vi "caluculator event structure.vi"() -> ()   [LabVIEW 2018]
panel:
  in  "stop":bool
  out "x/y":dbl
  out "x*y":dbl
  out "x-y":dbl
  out "C":dbl
  in  "B":dbl
  in  "A":dbl
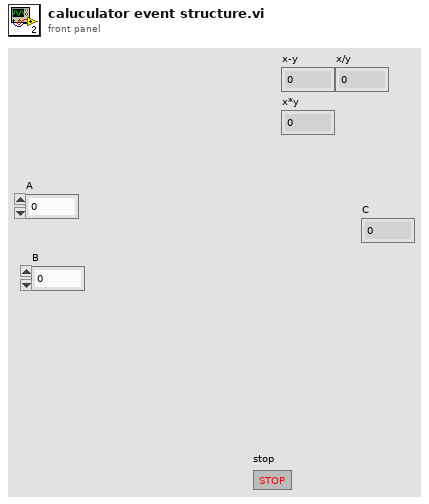
[diagram p1: front panel]
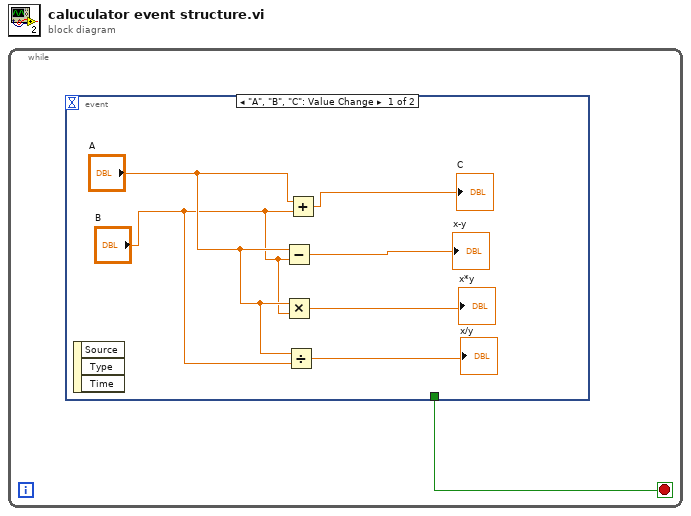
[diagram p0: block diagram]
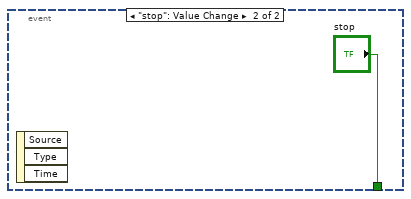
[diagram p2: hidden frame]
diagram:
  n1 = while {
    stop <- w1 stop-if-true
    n2 = event shown="[0] \"A\", \"B\", \"C\": Value Change" {
      selector: _ -> [_ _]
      dyn-events: _ -> [_ _]
      timeout: _ -> [_ _]
      tunnel: [_ "stop"] -> w1
      event "A", "B", "C": Value Change {
        n3 = event-data() -> ()  [unwired: 1 in, 3 out]
        n4 = Subtract(x="A", y="B") -> (x-y=→"x-y":dbl)
        n5 = Multiply(x="A", y="B") -> (x*y=→"x*y":dbl)
        n6 = Divide(x="A", y="B") -> (x/y=→"x/y":dbl)
        n7 = Add(x="A", y="B") -> (x+y=→"C":dbl)
      }
      event "stop": Value Change {
        n8 = event-data() -> ()  [unwired: 1 in, 3 out]
      }
    }
  }
